vi "ADCP_UI_Receive_List_Data_Packets.vi"() -> ()   [LabVIEW 2017]
panel:
  in  "Receive List Table Contents":string[][](array[string])
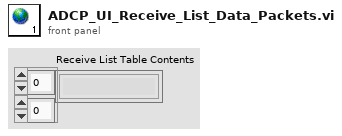
[diagram p1: front panel]
diagram:
